vi "Register gRPC Parameters.vi"(8 "error in (no error)":errorcluster, 11 "OOP Server in":refnum<class "OCVServer.lvclass">) -> (0 "error out":errorcluster, 3 "OOP Server out":refnum<class "OCVServer.lvclass">)   [LabVIEW 2019, in "OCVServer.lvlib" / "OCVServer.lvclass"]
uses:
  OCVServer.lvclass
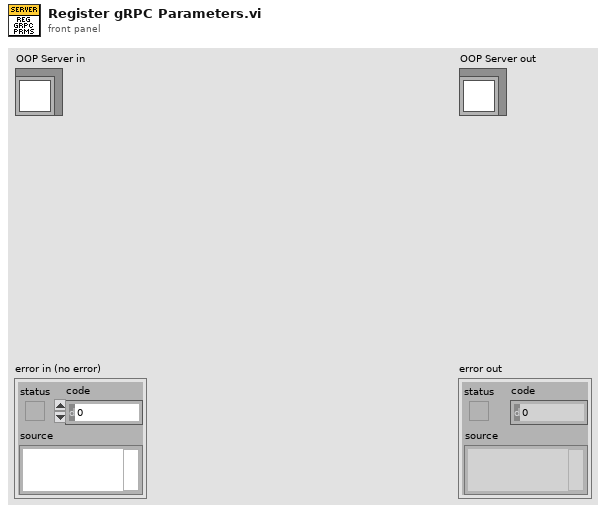
[diagram p1: front panel]
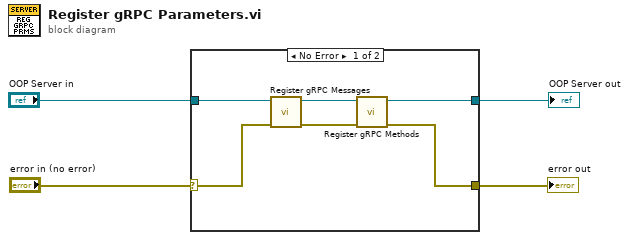
[diagram p0: block diagram]
diagram:
  n1 = case shown="No Error" "error in (no error)" {
    selector: "error in (no error)" -> [w8 w12]
    tunnel: [w6 w12] -> w3
    tunnel: [w10 w11] -> w1
    tunnel: "OOP Server in" -> [w9 w11]
    frame No Error {
      n2 = call "Register gRPC Messages.vi"("error in (no error)"=w8, "Template Server in"=w9) -> ("error out"=w7:errorcluster, "Template Server out"=w5:refnum<class "OCVServer.lvclass">)  [unwired: 8 in]
      n3 = call "Register gRPC Methods.vi"("error in (no error)"=w7, "Template Server in"=w5) -> ("error out"=w6:errorcluster, "Template Server out"=w10:refnum<class "OCVServer.lvclass">)  [unwired: 8 in]
    }
    frame Error {
    }
  }
  "error out" <- w3
  "OOP Server out" <- w1
